vi "globalTearDown.vi"(8 "error in (no error)":errorcluster, 11 "testcase-CSMArgument in":refnum<class "testcase-CSMArgument.lvclass">) -> (0 "error out":errorcluster, 3 "testcase-CSMArgument out":refnum<class "testcase-CSMArgument.lvclass">)   [LabVIEW 2017, in "testcase-CSMArgument.lvclass"]
uses:
  testcase-CSMArgument.lvclass
  testcase-CSMArgument.lvclass/testcase-CSMArgument.ctl
  <vilib>/addons/_JKI Toolkits/VI Tester/TestCase.llb/TestCase.lvclass
  src/user.lib/_NEVSTOP/Communicable State Machine(CSM)/Communicable State Machine.lvlib
  src/user.lib/_NEVSTOP/Communicable State Machine(CSM)/_Support/Typedef/_CSM_List Module Scope.ctl
panel:
  out "CSMs":string[](array[string])
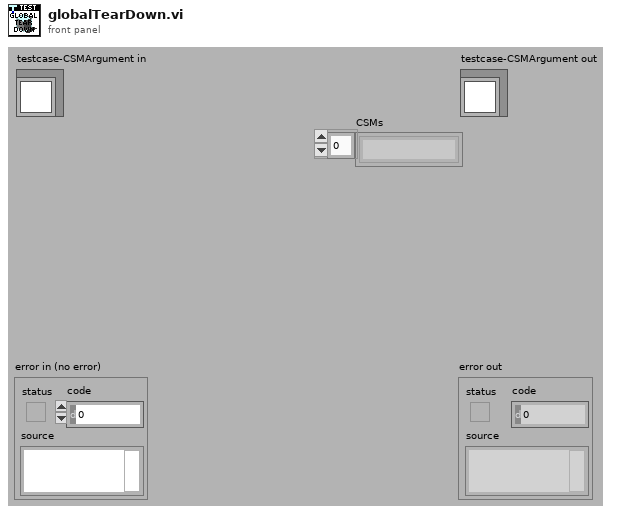
[diagram p1: front panel]
types:
  T1 = typedef "Communicable State Machine.lvlib/_CSM_List Module Scope.ctl" = enum16{"Normal", "System Only", "All"}
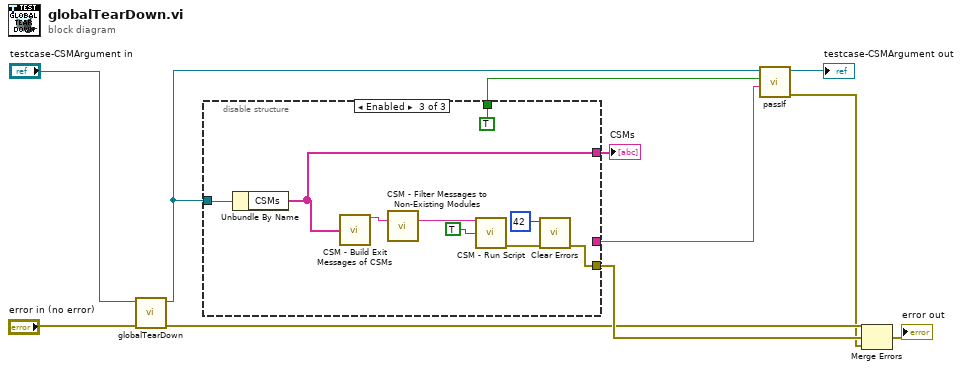
[diagram p0: block diagram]
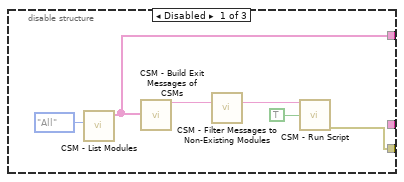
[diagram p2: hidden frame]
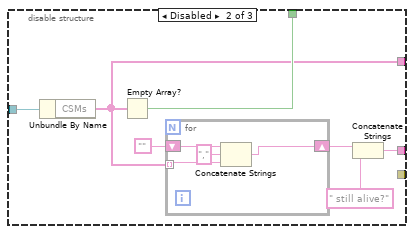
[diagram p3: hidden frame]
diagram:
  n1 = call-parent "globalTearDown.vi"("error in (no error)"="error in (no error)", "TestCase in"="testcase-CSMArgument in") -> ("error out"=w8:errorcluster, "TestCase out"=w5:refnum<class "testcase-CSMArgument.lvclass">)  [unwired: 8 in]
  n2 = disable-structure shown="Enabled" {
    disable-tunnel: [w13 _ w30] -> w10
    disable-tunnel: w5 -> [_ w24 w37]
    disable-tunnel: [w12 w22 w33] -> w1
    disable-tunnel: [_ w23 TRUE ("pass")] -> w3
    disable-tunnel: [_ w18 _] -> w2
    frame Disabled {
      n3 = call "CSM - List Modules.vi"("Scope (Normal)"=_CSM_List_Module_Scope."All") -> ("Module Names"=w12:string[])  [unwired: 9 in, 1 out]
      n4 = call "CSM - Build Exit Messages of CSMs.vi"("CSMs"=w12) -> ("States"=w17:string)  [unwired: 14 in]
      n5 = call "CSM - Filter Messages to Non-Existing Modules.vi"("States In"=w17) -> ("States Out"=w15:string)  [unwired: 14 in]
      n6 = call "CSM - Run Script.vi"("CSM Scripts"=w15, "Continue If Error? (F)"=TRUE) -> ("error out"=w13:errorcluster)  [unwired: 11 in, 2 out]
    }
    frame Disabled {
      n7 = Unbundle By Name(w24) -> ("CSMs"=w22:string[])
      n8 = Empty Array?(array=w22) -> (empty?=w23:bool)
      n9 = for {
        tunnel: w22 -> [w26] mode=indexing
        shift-right: [w27] -> w20
        shift-left: "" -> [w28]
        n10 = Concatenate Strings(w28, "," ("string"), w26) -> (w27:string)
      }
      n11 = Concatenate Strings(w20, " still alive?" ("string")) -> (w18:string)
    }
    frame Enabled {
      n12 = Unbundle By Name(w37) -> ("CSMs"=w33:string[])
      n13 = call "CSM - Build Exit Messages of CSMs.vi"("CSMs"=w33) -> ("States"=w36:string)  [unwired: 14 in]
      n14 = call "CSM - Filter Messages to Non-Existing Modules.vi"("States In"=w36) -> ("States Out"=w34:string)  [unwired: 14 in]
      n15 = call "CSM - Run Script.vi"("CSM Scripts"=w34, "Continue If Error? (F)"=TRUE) -> ("error out"=w32:errorcluster)  [unwired: 11 in, 2 out]
      n16 = call <vilib>:"Clear Errors.vi"("error in (no error)"=w32, "specific error code to clear (0: all)"=42) -> ("error out"=w30:errorcluster)  [unwired: 4 in, 1 out]
    }
  }
  "CSMs" <- w1
  n17 = call-dynamic "passIf.vi"("message (\"\")"=w2, "pass"=w3, "TestCase in"=w5) -> ("error out"=w4:errorcluster, "TestCase out"=→"testcase-CSMArgument out":refnum<class "testcase-CSMArgument.lvclass">)  [unwired: 7 in]
  n18 = Merge Errors(w8, w10, w4) -> (→"error out":errorcluster)
